vi "Get_ID.vi"(8 "error in (no error)":errorcluster, 11 "connection ID":refnum<k5>) -> (0 "error out":errorcluster, 2 "All ID list":u32[](array[numeric]) format="%x", 3 "connection ID out":refnum<k5>, 4 "Answer":string)   [LabVIEW 2015, in "VIPM2.lvlib"]
uses:
  VIPM2.lvlib
panel:
  # "GET ID"
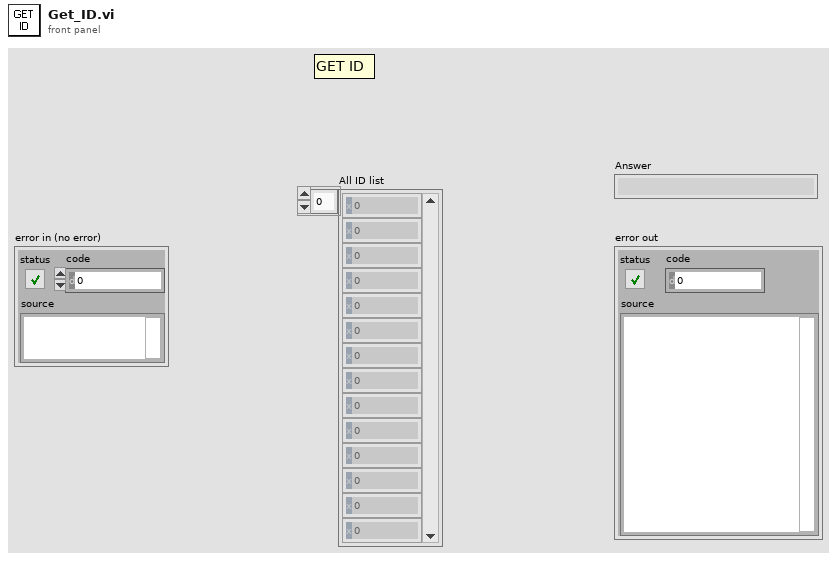
[diagram p1: front panel]
types:
  T1 = enum16{"Standard", "Buffered", "CRLF", "Immediate"}
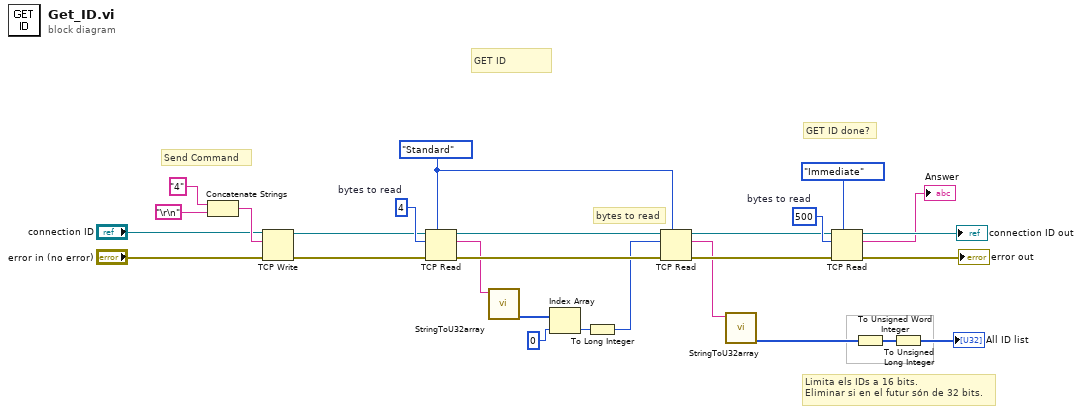
[diagram p0: block diagram]
diagram:
  w13 = 500  # bytes to read
  w18 = 4  # bytes to read
  w19 = T1."Standard" ("mode (standard)")
  # "Limita els IDs a 16 bits.\nEliminar si en el futur són de 32 bits."
  # "GET ID done?"
  # "bytes to read"
  # "GET ID"
  # "Send Command"
  n1 = Concatenate Strings("4" ("string"), "\r\n") -> (w25:string)
  n2 = TCP Write(connection ID="connection ID", data in=w25, error in (no error)="error in (no error)") -> (connection ID out=w17:refnum<k5>, error out=w16:errorcluster)  [unwired: 1 in, 1 out]
  n3 = TCP Read(connection ID=w17, bytes to read=w18, error in (no error)=w16, 7:w19) -> (connection ID out=w22:refnum<k5>, data out=w15:string, error out=w21:errorcluster)  [unwired: 1 in]
  n4 = call "StringToU32array.vi"("String"=w15) -> ("U32array"=w14:u32[])  [unwired: 2 out]
  n5 = Index Array "Index Array"(array=w14, index=0) -> (element=w5:u32)
  n6 = To Long Integer(number=w5) -> (32bit integer=w4:i32)
  n7 = TCP Read(connection ID=w22, bytes to read=w4, error in (no error)=w21, 7:w19) -> (connection ID out=w11:refnum<k5>, data out=w6:string, error out=w10:errorcluster)  [unwired: 1 in]
  n8 = call "StringToU32array.vi"("String"=w6) -> ("U32array"=w2:u32[])  [unwired: 2 out]
  n9 = TCP Read(connection ID=w11, bytes to read=w13, error in (no error)=w10, 7:T1."Immediate" ("mode (standard)")) -> (connection ID out=→"connection ID out":refnum<k5>, data out=→"Answer":string, error out=→"error out":errorcluster)  [unwired: 1 in]
  n10 = To Unsigned Word Integer(number=w2) -> (unsigned 16bit integer=w3:u16[])
  n11 = To Unsigned Long Integer(number=w3) -> (unsigned 32bit integer=→"All ID list":u32[])
